vi "is module blocking.vi"(8 "error in":errorcluster, 11 "module configuration in":refnum<class "TBM module configuration.lvclass">) -> (0 "error out":errorcluster, 2 "module timing":T1, 3 "module configuration out":refnum<class "TBM module configuration.lvclass">)   [LabVIEW 2013, in "TBM module configuration.lvclass"]
doc: "Modules are usually intended to be non-blocking, but in some cases they abstract APIs which are known to be non-deterministic. This property indicates the determinism of the module.\n\nDeterministic - No shared resources, no parallel code execution, no memory allocation etc. This is the best-case in terms of execution. Example: Scaling function, pure processing, etc.\n\nNon-blocking - The code is guaranteed to return quickly, but may not be strictly deterministic. Examples: CVT, OPC UA slave, Modbus slave\n\nBlocking - The function is not guaranteed to return quickly or guaranteed to not return quickly. Example: Modbus master, OPC UA client\n\nIn some cases the module is implemented in such a way to make the module deterministic even if the API is not. For example, the current TDMS logger implementation is deterministic."
uses:
  TBM module configuration.lvclass
  module execution time property.ctl
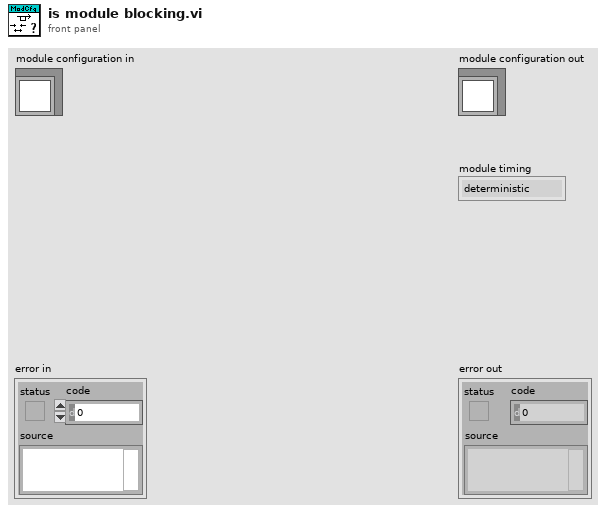
[diagram p1: front panel]
types:
  T1 = typedef "TBM module configuration.lvclass/module execution time property.ctl" = enum16{"deterministic", "non-blocking", "blocking"}
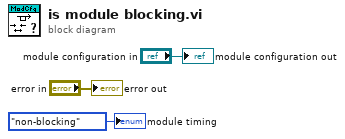
[diagram p0: block diagram]
diagram:
  "error out" <- "error in"
  "module configuration out" <- "module configuration in"
  "module timing" <- module_execution_time_property."non-blocking" ("module timing")
